vi "svm_load_model.vi"(8 "error in (no error)":errorcluster, 11 "File path":path) -> (0 "error out":errorcluster, 3 "Model":T1)   [LabVIEW 2014]
uses:
  Controls/svm_model.ctl
  Controls/svm_parameter.ctl
  Controls/svm_type.ctl
  Controls/svm_kernel_type.ctl
  Controls/svm_node.ctl
  bin/x64/LVLibSVM.dll
  Controls/svm_node_padded.ctl
  Controls/svm_model_padded.ctl
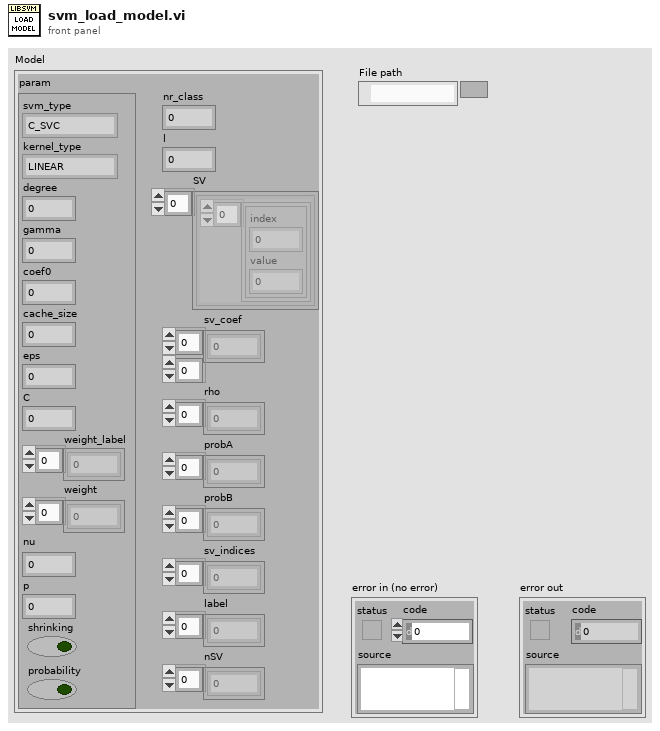
[diagram p1: front panel]
types:
  T1 = typedef "svm_model.ctl" = cluster{"param":T2, "nr_class":i32, "l":i32, "SV":cluster{"Array":T5[]}[], "sv_coef":dbl[][], "rho":dbl[], "probA":dbl[], "probB":dbl[], "sv_indices":i32[], "label":i32[], "nSV":i32[]}
  T2 = typedef "svm_parameter.ctl" = cluster{"svm_type":T3, "kernel_type":T4, "degree":i32, "gamma":dbl, "coef0":dbl, "cache_size":dbl, "eps":dbl, "C":dbl, "weight_label":i32[], "weight":dbl[], "nu":dbl, "p":dbl, "shrinking":bool, "probability":bool}
  T3 = typedef "svm_type.ctl" = enum32{"C_SVC", "NU_SVC", "ONE_CLASS", "EPSILON_SVR", "NU_SVR"}
  T4 = typedef "svm_kernel_type.ctl" = enum32{"LINEAR", "POLY", "RBF", "SIGMOID", "PRECOMPUTED"}
  T5 = typedef "svm_node.ctl" = cluster{"index":i32, "value":dbl}
  T6 = typedef "svm_model_padded.ctl" = cluster{"param":T2, "nr_class":i32, "l":i32, "SV":cluster{"Array":T7[]}[], "sv_coef":dbl[][], "rho":dbl[], "probA":dbl[], "probB":dbl[], "sv_indices":i32[], "label":i32[], "nSV":i32[]}
  T7 = typedef "svm_node_padded.ctl" = cluster{"index":i32, "padding":i32, "value":dbl}
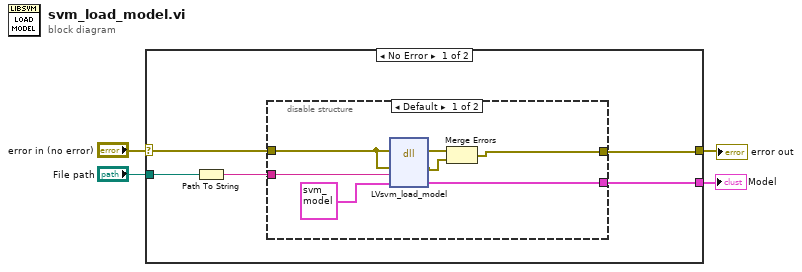
[diagram p0: block diagram]
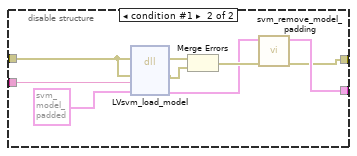
[diagram p2: hidden frame]
diagram:
  n1 = case shown="No Error" "error in (no error)" {
    selector: "error in (no error)" -> [w7 w26]
    tunnel: [w6 w26] -> w4
    tunnel: "File path" -> [w9 _]
    tunnel: [w5 _] -> w1
    frame No Error {
      n2 = Path To String(path=w9) -> (string=w8:string)
      n3 = disable-structure shown="Default" {
        disable-tunnel: w8 -> [w16 w25]
        disable-tunnel: w7 -> [w15 w24]
        disable-tunnel: [w12 w17] -> w6
        disable-tunnel: [w11 w19] -> w5
        frame condition #0 (active) {
          n4 = dll-call lib="C:/dev/LabVIEW-libsvm/LabVIEW/bin/x64/LVLibSVM.*" fn="LVsvm_load_model"(error in=w15, "lvErr"=w15, "path_in"=w16, T1 {"param"={"svm_type"=enum."C_SVC", "kernel_type"=enum."LINEAR", "degree"=0, "gamma"=0.0, "coef0"=0.0, "cache_size"=0.0, "eps"=0.0, "C"=0.0, "weight_label"=[], "weight"=[], "nu"=0.0, "p"=0.0, "shrinking"=FALSE, "probability"=FALSE}, "nr_class"=0, "l"=0, "SV"=[], "sv_coef"=[], "rho"=[], "probA"=[], "probB"=[], "sv_indices"=[], "label"=[], "nSV"=[]} ("svm_model")) -> (error out=w14:errorcluster, "lvErr"=w13:errorcluster, w11:T1)  [unwired: 4 in, 1 out]
          n5 = Merge Errors(w14, w13) -> (w12:errorcluster)
        }
        frame condition #1 {
          n6 = dll-call lib="C:/dev/LabVIEW-libsvm/LabVIEW/bin/x64/LVLibSVM.*" fn="LVsvm_load_model"(error in=w24, "lvErr"=w24, "path_in"=w25, "Padded model"=T6 {"param"={"svm_type"=enum."C_SVC", "kernel_type"=enum."LINEAR", "degree"=0, "gamma"=0.0, "coef0"=0.0, "cache_size"=0.0, "eps"=0.0, "C"=0.0, "weight_label"=[], "weight"=[], "nu"=0.0, "p"=0.0, "shrinking"=FALSE, "probability"=FALSE}, "nr_class"=0, "l"=0, "SV"=[], "sv_coef"=[], "rho"=[], "probA"=[], "probB"=[], "sv_indices"=[], "label"=[], "nSV"=[]} ("svm_model")) -> (error out=w23:errorcluster, "lvErr"=w22:errorcluster, "Padded model"=w20:T6)  [unwired: 4 in, 1 out]
          n7 = Merge Errors(w23, w22) -> (w21:errorcluster)
          n8 = call "svm_remove_model_padding.vi"("error in (no error)"=w21, "Padded model"=w20) -> ("error out"=w17:errorcluster, "Model"=w19:T1)  [unwired: 8 in]
        }
      }
    }
    frame Error {
    }
  }
  "error out" <- w4
  "Model" <- w1
